vi "Write module boolean values.vi"(9 "Label.Text":string="Phase Shift, deg", 10 "data (T)":bool=TRUE, 11 "module ref":refnum<vi>) -> ()   [LabVIEW 2017]
panel:
  out "Boolean Ref":refnum<vi>
  out "error out":errorcluster
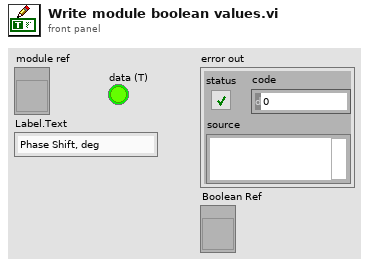
[diagram p1: front panel]
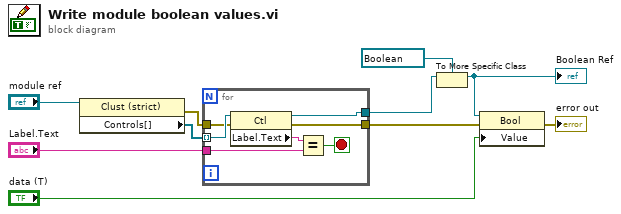
[diagram p0: block diagram]
diagram:
  n1 = property class="Clust (strict)"(reference="module ref") -> (error out=w4:errorcluster, "Controls[]"=w10:refnum<vi>[])  [unwired: 1 in, 1 out]
  n2 = for {
    tunnel: w10 -> [w17] mode=indexing
    tunnel: "Label.Text" -> [w16]
    tunnel: [w13] -> w8
    tunnel: w4 -> [w12]
    tunnel: [w11] -> w3
    stop <- w14 stop-if-true
    n3 = property class="Ctl"(reference=w17, error in=w12) -> (reference out=w13:refnum<vi>, error out=w11:errorcluster, "Label.Text"=w15:string)
    n4 = Equal?(x=w15, y=w16) -> (x = y?=w14:bool)
  }
  n5 = To More Specific Class(target class=refnum<vi> refnum ("Phase Shift, deg"), reference=w8) -> (specific class reference=w6:refnum<vi>)  [unwired: 1 in, 1 out]
  "Boolean Ref" <- w6
  n6 = property class="Bool"(reference=w6, error in=w3, "Value"="data (T)") -> (error out=→"error out":errorcluster)  [unwired: 1 out]
